vi "Auton List.vi"() -> (3 "String Array":string[](array[string]))   [LabVIEW 2018]
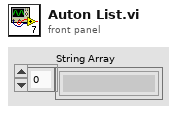
[diagram p1: front panel]
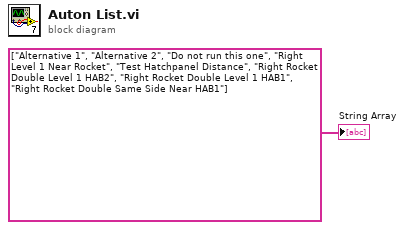
[diagram p0: block diagram]
diagram:
  "String Array" <- string[] ["Alternative 1", "Alternative 2", "Do not run this one", "Right Level 1 Near Rocket", "Test Hatchpanel Distance", "Right Rocket Double Level 1 HAB2", "Right Rocket Double Level 1 HAB1", "Right Rocket Double Same Side Near HAB1"] ("String Array")
